vi "ATF-Hardware Config.vi"() -> ()   [LabVIEW 2022 SP3]
uses:
  Controls/SeCrTs-Config.ctl
panel:
  in  "Signal list":bool
  out "Config":T1={"AO config"=[], "AI config"=[], "DI config"=[], "DO config"=[], "TC config"=[{"Channel_Name"="", "Channel_Number"="", "Pre_Scale_min"=0.0, "Pre_Scale_max"=0.0, "units"=4, " type"=7}], "ACC config"=[], "SG config"=[], "Strain Gauge Settings"={"poisson ratio"=0.3, "nominal gage resistance"=120.0, "gage factor"=2.08}, "Bridge Settings"={"voltage excitation value"=3.3, "voltage excitation source"=10200, "initial bridge voltage"=0.0, "lead wire resistance"=1.7, "strain configuration"=10271}, "Sample Rate"={"AI Sample Rate"=[], "AO Sample Rate"=[], "DI Sample Rate"=[], "TC Sample Rate"=[], "DO Sample Rate"=[], "SG Sample Rate"=[], "ACC Sample Rate"=[]}} {"Bridge Settings"."strain configuration" items=["Full Bridge I"=10183, "Full Bridge II"=10184, "Full Bridge III"=10185, "Half Bridge I"=10188, "Half Bridge II"=10189, "Quarter Bridge I"=10271, "Quarter Bridge II"=10272]; "Bridge Settings"."voltage excitation source" items=["Internal"=10200, "External"=10167, "None"=10230]; "ACC config"."Terminal configuration" items=["default"=-1, "RSE"=10083, "NRSE"=10078, "Differential"=10106, "Pseudodifferential"=12529]; "ACC config"."Sensitivity units" items=["mVolts/g"=12509, "Volts/g"=12510]; "TC config"."type" items=["J"=10072, "K"=10073, "N"=10077, "R"=10082, "S"=10085, "T"=10086, "B"=10047, "E"=10055]; "TC config"."units" items=["Deg C", "Deg F", "Kelvins", "Deg R", "From Custom Scale"]}
  in  "Cancel":bool
  in  "Load Configuration":bool
  in  "New configuration":bool
  in  "Save Config":bool
  in  "Tab Control":T2(tab)
  in  "DO Sample Rate":dbl[](array[numeric]) format="%#_g Hz"
  in  "DO config":T3(array[cluster])=[{"Channel_Name"="", "Channel_Number"="", "Default_Value"=FALSE, "Units"=FALSE}]
  out "DO Device List":string[](array[string])
  in  "DI Sample Rate":dbl[](array[numeric]) format="%#_g Hz"
  in  "DI config":T3(array[cluster])
  out "DI Device List":string[](array[string])
  in  "AO Sample Rate":dbl[](array[numeric]) format="%#_g Hz"
  in  "AO config":T4(array[cluster])
  out "AO Device List":string[](array[string])
  in  "AI Sample Rate":dbl[](array[numeric]) format="%#_g Hz"
  in  "AI config":T5(array[cluster])
  out "AI Device List":string[](array[string])
  in  "TC Sample Rate":dbl[](array[numeric]) format="%#_g Hz"
  in  "TC config":T6(array[cluster]) {"thermocouple type" items=["J"=10072, "K"=10073, "N"=10077, "R"=10082, "S"=10085, "T"=10086, "B"=10047, "E"=10055]; "units" items=["Deg C"=10143, "Deg F"=10144, "Kelvins"=10325, "Deg R"=10145, "From Custom Scale"=10065]}
  out "TC Device List":string[](array[string])
  in  "ACC Sample Rate":dbl[](array[numeric]) format="%#_g Hz"
  in  "ACC config":T7(array[cluster]) {"Sensitivity units" items=["mVolts/g"=12509, "Volts/g"=12510]; "Terminal configuration" items=["default"=-1, "RSE"=10083, "NRSE"=10078, "Differential"=10106, "Pseudodifferential"=12529]}
  out "ACC Device List":string[](array[string])
  out "SG Device List":string[](array[string])
  in  "SG Sample Rate":dbl[](array[numeric]) format="%#_g Hz"
  in  "SG config":T8(array[cluster])
  in  "SG Settings":T9={"gage factor"=2.08, "nominal gage \nresistance"=120.0, "poisson ratio"=0.3}
  in  "Bridge Settings":T10={"voltage excitation value"=3.3, "voltage excitation source"=10200, "initial bridge voltage"=0.0, "lead wire resistance"=1.7, "strain configuration"=10271} {"strain configuration" items=["Full Bridge I"=10183, "Full Bridge II"=10184, "Full Bridge III"=10185, "Half Bridge I"=10188, "Half Bridge II"=10189, "Quarter Bridge I"=10271, "Quarter Bridge II"=10272]; "voltage excitation source" items=["Internal"=10200, "External"=10167, "None"=10230]}
  # "DO_Channel_Name"
  # "DO_Channel_Number"
  # "Default Value"
  # "Invert?"
  # "DI_Channel_Name"
  # "DI_Channel_Number"
  # "Default Value"
  # "Invert?"
  # "AO_Channel_Name"
  # "AO_Channel_Number"
  # "Default Value"
  # "Units"
  # "AI_Channel_Name"
  # "AI_Channel_Number"
  # "Pre_Scale_min"
  # "Pre_Scale_max"
  # "Scale_min"
  # "Scale_max"
  # "Units"
  # "TC_Channel_Name"
  # "TC_Channel_Number"
  # "Max_Value"
  # "Units"
  # "Type"
  # "Min_Value"
  # "ACC_Channel_Name"
  # "ACC_Channel_Number"
  # "Min_Value"
  # "Max_Value"
  # "Terminal Config"
  # "Sensitivity"
  # "Sensitivity Units"
  # "SG_Channel_Name"
  # "SG_Channel_Number"
  # "Min_Value"
  # "Max_Value"
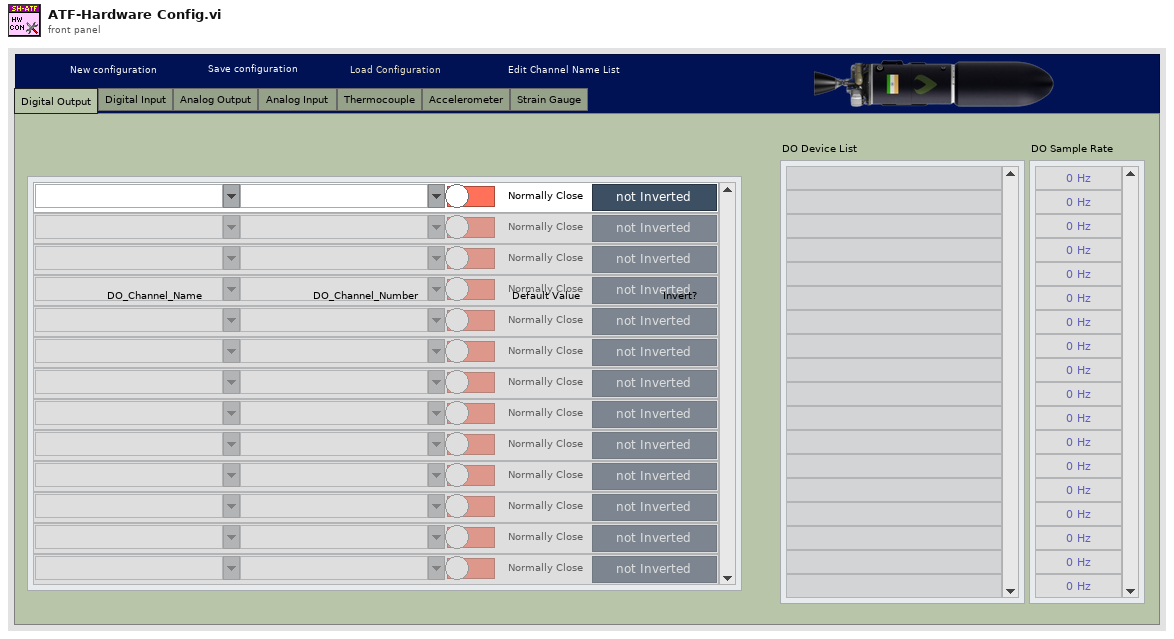
[diagram p1: front panel]
types:
  T1 = typedef "SeCrTs-Config.ctl" = cluster{"AO config":cluster{"Channel_Name":string, "Channel_Number":string, "Default_Value":dbl, "Units":string}[], "AI config":cluster{"Channel_Name":string, "Channel_Number":string, "Pre_Scale_min":dbl, "Pre_Scale_max":dbl, "Sensor_min":dbl, "Sensor_max":dbl, "Units":string}[], "DI config":cluster{"Channel_Name":string, "Channel_Number":string, "Default_Value":bool, "DI invert?":bool}[], "DO config":cluster{"Channel_Name":string, "Channel_Number":string, "Default_Value":bool, "DO invert?":bool}[], "TC config":cluster{"Channel_Name":string, "Channel_Number":string, "Pre_Scale_min":dbl, "Pre_Scale_max":dbl, "units":i32, " type":i32}[], "ACC config":cluster{"Channel_Name":string, "Channel_Number":string, "Pre_Scale_min":dbl, "Pre_Scale_max":dbl, "Terminal configuration":i32, "Sensitivity":dbl, "Sensitivity units":i32}[], "SG config":cluster{"Channel_Name":string, "Channel_Number":string, "Pre_Scale_min":dbl, "Pre_Scale_max":dbl}[], "Strain Gauge Settings":cluster{"poisson ratio":dbl, "nominal gage resistance":dbl, "gage factor":dbl}, "Bridge Settings":cluster{"voltage excitation value":dbl, "voltage excitation source":i32, "initial bridge voltage":dbl, "lead wire resistance":dbl, "strain configuration":i32}, "Sample Rate":cluster{"AI Sample Rate":dbl[], "AO Sample Rate":dbl[], "DI Sample Rate":dbl[], "TC Sample Rate":dbl[], "DO Sample Rate":dbl[], "SG Sample Rate":dbl[], "ACC Sample Rate":dbl[]}}
  T2 = enum32{"Digital Output", "Digital Input", "Analog Output", "Analog Input ", "Thermocouple", "Accelerometer", "Strain Gauge"}
  T3 = cluster{"Channel_Name":string, "Channel_Number":string, "Default_Value":bool, "Units":bool}[]
  T4 = cluster{"Channel_Name":string, "Channel_Number":string, "Default_Value":dbl, "Units":string}[]
  T5 = cluster{"Channel_Name":string, "Channel_Number":string, "Pre_Scale_min":dbl, "Pre_Scale_max":dbl, "Sensor_min":dbl, "Sensor_max":dbl, "Units":string}[]
  T6 = cluster{"Channel_Name":string, "Channel_Number":string, "Pre_Scale_min":dbl, "Pre_Scale_max":dbl, "units":i32, "thermocouple type":i32}[]
  T7 = cluster{"Channel_Name":string, "Channel_Number":string, "Pre_Scale_min":dbl, "Pre_Scale_max":dbl, "Terminal configuration":i32, "Sensitivity":dbl, "Sensitivity units":i32}[]
  T8 = cluster{"Channel_Name":string, "Channel_Number":string, "Pre_Scale_min":dbl, "Pre_Scale_max":dbl}[]
  T9 = cluster{"gage factor":dbl, "nominal gage \nresistance":dbl, "poisson ratio":dbl}
  T10 = cluster{"voltage excitation value":dbl, "voltage excitation source":i32, "initial bridge voltage":dbl, "lead wire resistance":dbl, "strain configuration":i32}
  T11 = cluster{"Device List":cluster{"AO Cards":tag[], "AI Cards":tag[], "DI Cards":tag[], "DO Cards":tag[]}, "Channel List":cluster{"AI Channel list":tag[], "AO Channel list":tag[], "DO Channel list ":tag[], "DI Channel list":tag[]}}
  T12 = cluster{"Channel List":cluster{"AI Channel list":tag[], "AO Channel list":tag[], "DO Channel list ":tag[], "DI Channel list":tag[]}, "Device List":cluster{"AO Cards":tag[], "AI Cards":tag[], "DI Cards":tag[], "DO Cards":tag[]}}
  T13 = cluster{"Data":T1, "path":path, "Name ref":refnum<vi>[], "Names":string[][], "Signal path":path, "SR":cluster{"AI Sample Rate":dbl[], "AO Sample Rate":dbl[], "DI Sample Rate":dbl[], "TC Sample Rate":dbl[], "DO Sample Rate":dbl[], "SG Sample Rate":dbl[], "ACC Sample Rate":dbl[]}, "Device List":cluster{"AO Cards":tag[], "AI Cards":tag[], "DI Cards":tag[], "DO Cards":tag[]}}
  T14 = typedef "SeCrTs-file folder ctl.ctl" = cluster{"Datalog path":path, "Configuration path":path, "Signal list path":path, "Sub vi's":path, "Authentication":path, "Sequence":path, "Event Log":path, "CS Error log":path, "RT Error Log":path}
  T15 = cluster{"AI":string[], "DI":string[], "DO":string[], "SG":string[], "AO":string[], "TC":string[], "ACC":string[]}
  T16 = cluster{"AI Channel list":tag[], "AO Channel list":tag[], "DO Channel list ":tag[], "DI Channel list":tag[]}
  T17 = cluster{"AO Cards":tag[], "AI Cards":tag[], "DI Cards":tag[], "DO Cards":tag[]}
  T18 = cluster{"AI Sample Rate":dbl[], "AO Sample Rate":dbl[], "DI Sample Rate":dbl[], "TC Sample Rate":dbl[], "DO Sample Rate":dbl[], "SG Sample Rate":dbl[], "ACC Sample Rate":dbl[]}
  T19 = enum16{"open", "replace", "create", "open or create", "replace or create", "replace or create with confirmation"}
  T20 = enum32{"Invalid", "Standard", "Closed", "Hidden", "Minimized", "Maximized"}
  T21 = cluster{"Channel_Name":string, "Channel_Number":string, "Default_Value":bool, "DI invert?":bool}[]
  T22 = cluster{"Channel_Name":string, "Channel_Number":string, "Default_Value":bool, "DO invert?":bool}[]
  T23 = cluster{"Channel_Name":string, "Channel_Number":string, "Pre_Scale_min":dbl, "Pre_Scale_max":dbl, "units":i32, " type":i32}[]
  T24 = cluster{"poisson ratio":dbl, "nominal gage resistance":dbl, "gage factor":dbl}
  T25 = cluster{"Channel_Name":string, "Channel_Number":string}
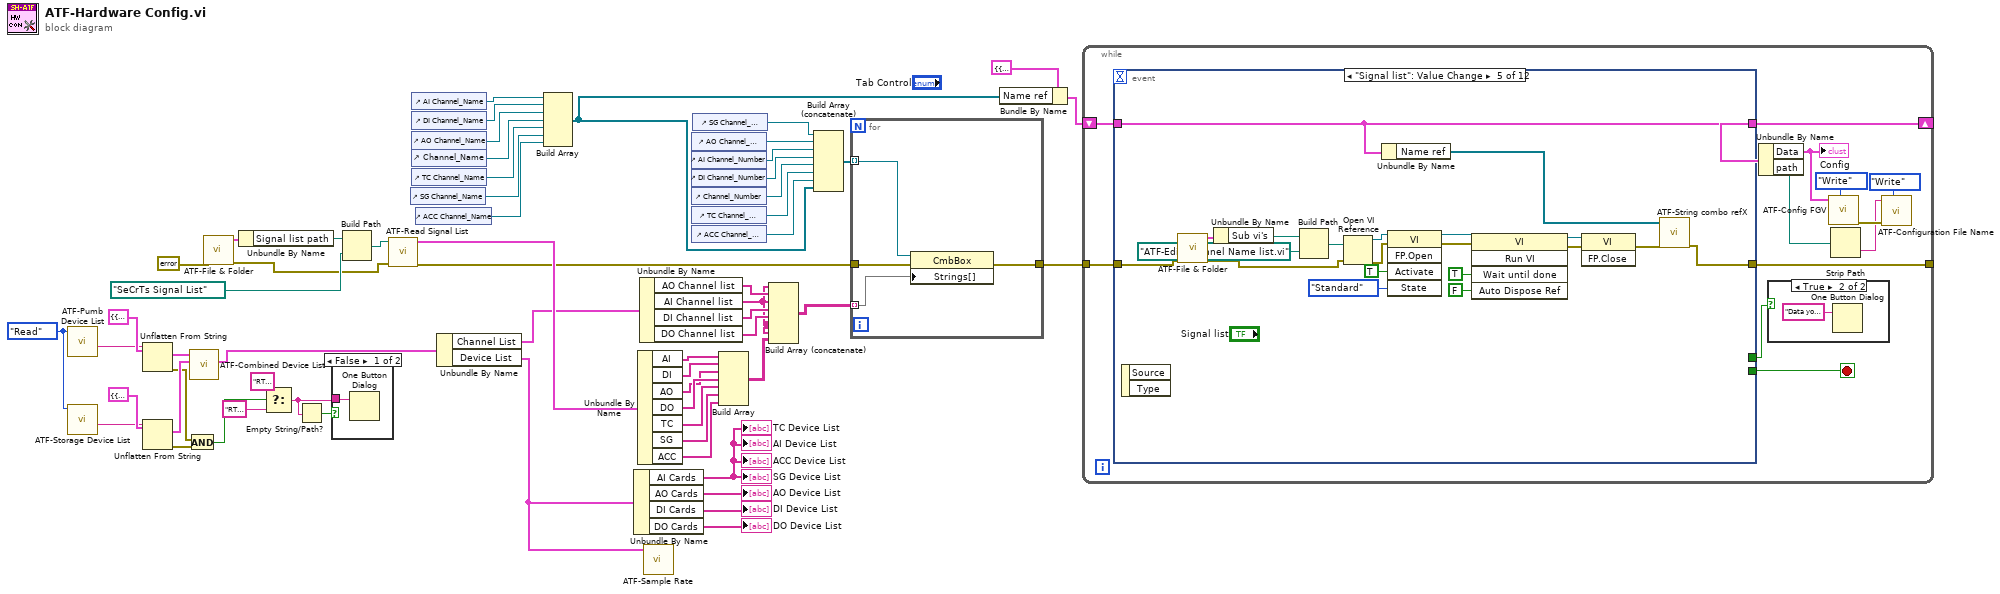
[diagram p0: block diagram]
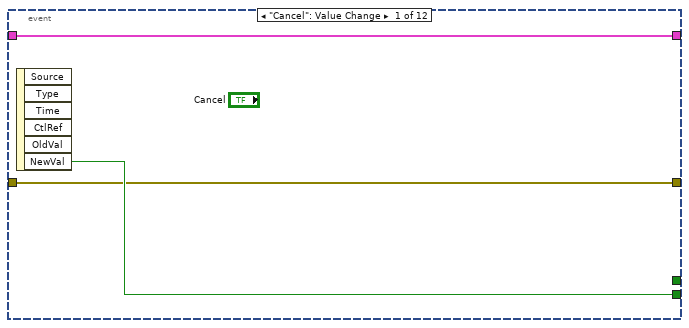
[diagram p4: hidden frame]
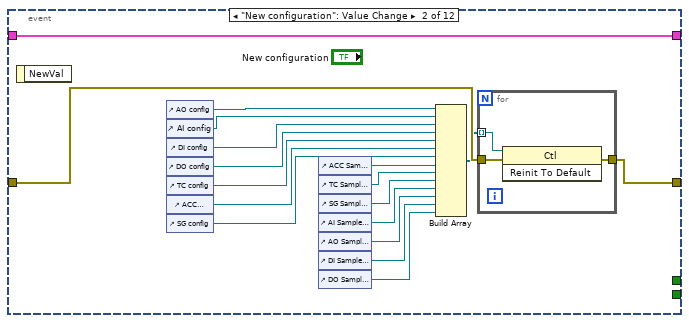
[diagram p5: hidden frame]
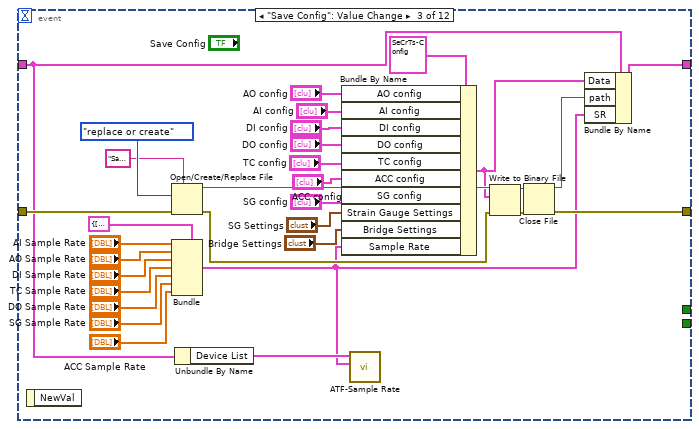
[diagram p6: hidden frame]
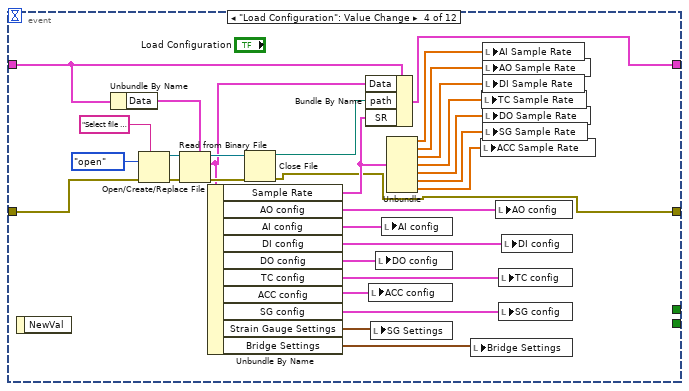
[diagram p7: hidden frame]
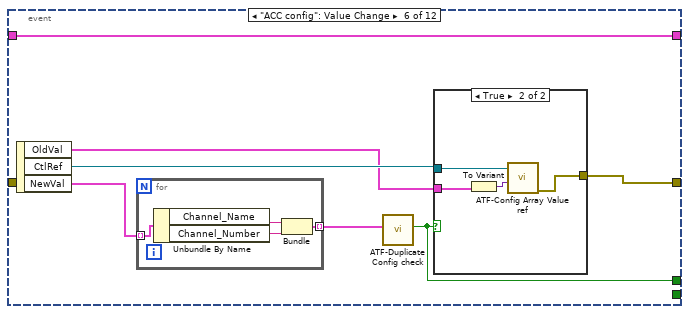
[diagram p8: hidden frame]
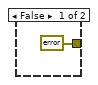
[diagram p9: hidden frame]
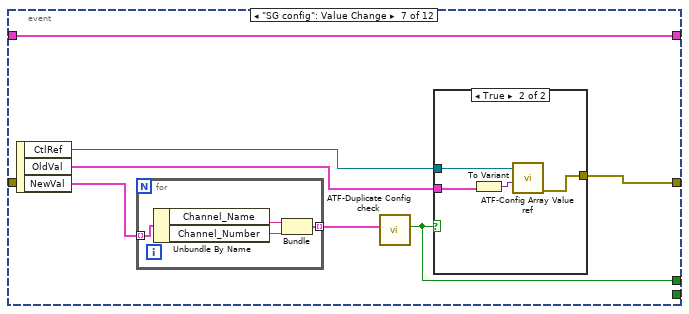
[diagram p10: hidden frame]
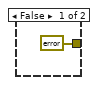
[diagram p11: hidden frame]
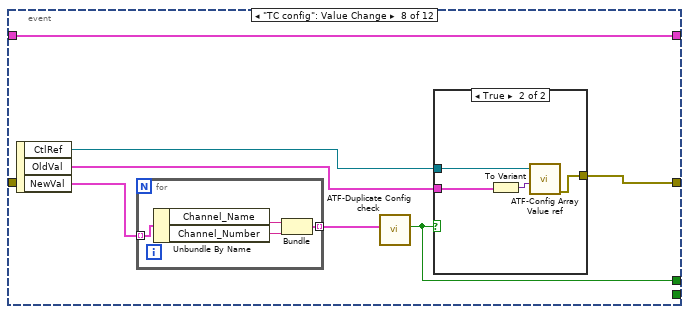
[diagram p12: hidden frame]
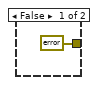
[diagram p13: hidden frame]
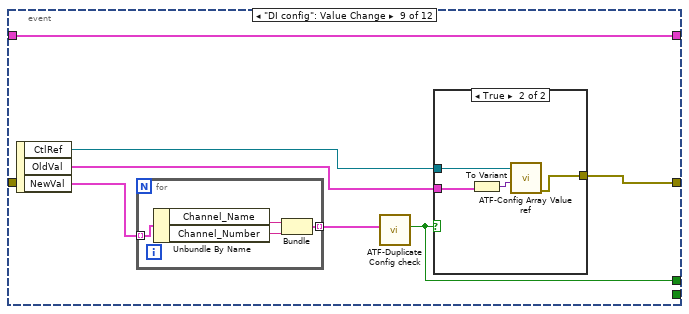
[diagram p14: hidden frame]
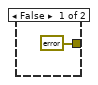
[diagram p15: hidden frame]
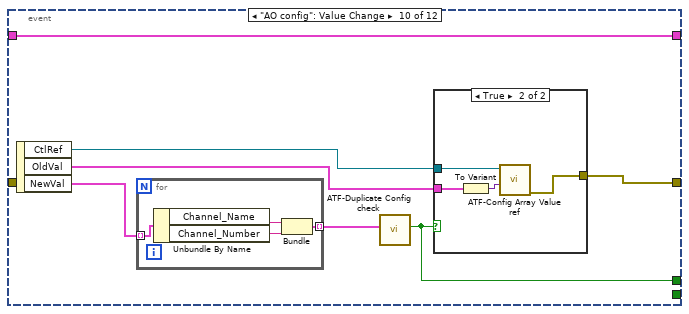
[diagram p16: hidden frame]
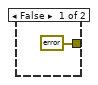
[diagram p17: hidden frame]
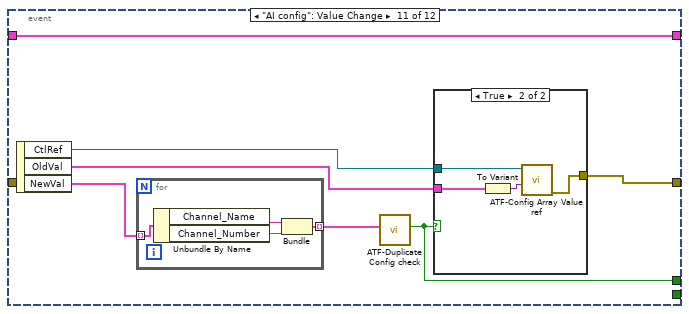
[diagram p18: hidden frame]
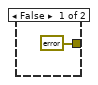
[diagram p19: hidden frame]
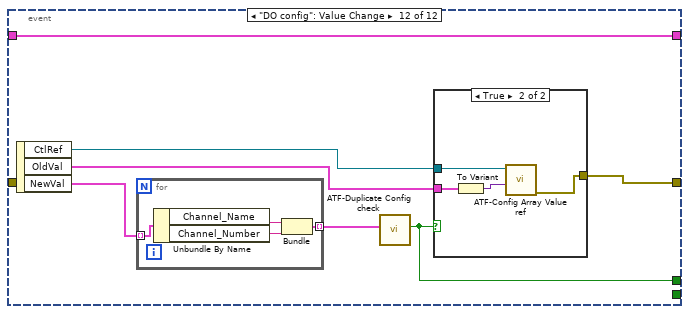
[diagram p20: hidden frame]
diagram:
  w14 = enum16{"Read", "Write", "Clear"}."Read" ("Enum")
  n1 = call "ATF-Pumb Device List.vi"("Enum"=w14) -> ("DL"=w3:string)  [unwired: 10 in]
  n2 = call "ATF-Storage Device List.vi"("Enum"=w14) -> ("DL"=w2:string)  [unwired: 10 in]
  n3 = Unflatten From String(type=T11 {"Device List"={"AO Cards"=[], "AI Cards"=[], "DI Cards"=[], "DO Cards"=[]}, "Channel List"={"AI Channel list"=[], "AO Channel list"=[], "DO Channel list "=[], "DI Channel list"=[]}}, binary string=w3) -> (value=w11:T11, error out=w6:errorcluster)  [unwired: 3 in, 1 out]
  n4 = Unflatten From String(type=T12 {"Channel List"={"AI Channel list"=[], "AO Channel list"=[], "DO Channel list "=[], "DI Channel list"=[]}, "Device List"={"AO Cards"=[], "AI Cards"=[], "DI Cards"=[], "DO Cards"=[]}}, binary string=w2) -> (value=w10:T12, error out=w5:errorcluster)  [unwired: 3 in, 1 out]
  n5 = And(x=w6, y=w5) -> (x .and. y?=w4:bool)
  n6 = call "ATF-Combined Device List.vi"("Storage"=w10, "Pump"=w11) -> ("Combined Device list"=w15:T12)  [unwired: 9 in]
  n7 = call "ATF-File & Folder.vi"("error in (no error)"=errorcluster {"status"=FALSE, "code"=0, "source"=""} ("error in")) -> ("error out"=w40:errorcluster, "File Output"=w46:T14)  [unwired: 9 in]
  n8 = Unbundle By Name(w46) -> ("Signal list path"=w45:path)
  n9 = Select(t="RT device list has not loaded!" ("DL"), s=w4, f="RT device list has been loaded.") -> (s? t:f=w7:string)
  n10 = Empty String/Path?(string/path=w7) -> (empty?=w9:bool)
  n11 = case shown="False" w9 {
    tunnel: w7 -> [w62 _]
    frame False {
      n12 = One Button Dialog(message=w62) -> ()  [unwired: 1 in, 1 out]
    }
    frame True {
    }
  }
  n13 = Build Path(base path=w45, name or relative path=path "SeCrTs Signal List") -> (appended path=w19:path)
  n14 = call "ATF-Read Signal List.vi"("error in"=w40, "file path (use dialog)"=w19) -> ("error out"=w18:errorcluster, "Names"=w39:T15)  [unwired: 8 in]
  n15 = control-ref of="SG Channel_Name"() -> (w25:refnum<vi>)
  n16 = control-ref of="AI Channel_Name"() -> (w43:refnum<vi>)
  n17 = control-ref of="DI Channel_Name"() -> (w42:refnum<vi>)
  n18 = control-ref of="AO Channel_Name"() -> (w27:refnum<vi>)
  n19 = control-ref of="Channel_Name"() -> (w26:refnum<vi>)
  n20 = control-ref of="TC Channel_Name"() -> (w41:refnum<vi>)
  n21 = control-ref of="ACC Channel_Name"() -> (w24:refnum<vi>)
  n22 = Unbundle By Name(w15) -> ("Channel List"=w16:T16, "Device List"=w17:T17)
  n23 = Build Array(w43, w42, w27, w26, w41, w25, w24) -> (w28:refnum<vi>[])
  n24 = Unbundle By Name(w17) -> ("AI Cards"=→"AI Device List" →"TC Device List" →"ACC Device List" →"SG Device List":tag[], "AO Cards"=→"AO Device List":tag[], "DI Cards"=→"DI Device List":tag[], "DO Cards"=→"DO Device List":tag[])
  n25 = Unbundle By Name(w39) -> ("AI"=w38:string[], "DI"=w37:string[], "AO"=w32:string[], "DO"=w36:string[], "TC"=w35:string[], "SG"=w34:string[], "ACC"=w33:string[])
  n26 = Unbundle By Name(w16) -> ("AO Channel list"=w49:tag[], "AI Channel list"=w48:tag[], "DI Channel list"=w56:tag[], "DO Channel list"=w55:tag[])
  n27 = call "ATF-Sample Rate.vi"("Device List"=w17) -> ()  [unwired: 11 in]
  n28 = control-ref of="AO Channel_Number"() -> (w61:refnum<vi>)
  n29 = control-ref of="AI Channel_Number"() -> (w60:refnum<vi>)
  n30 = control-ref of="DI Channel_Number"() -> (w59:refnum<vi>)
  n31 = control-ref of="Channel_Number"() -> (w58:refnum<vi>)
  n32 = control-ref of="TC Channel_Number"() -> (w52:refnum<vi>)
  n33 = control-ref of="ACC Channel_Number"() -> (w51:refnum<vi>)
  n34 = control-ref of="SG Channel_Number"() -> (w50:refnum<vi>)
  n35 = Build Array(w38, w37, w32, w36, w35, w34, w33) -> (w31:string[][])
  n36 = Build Array (concatenate)(w48, w49, w48, w56, w55, w48, w48, w31) -> (w54:string[][])
  n37 = Build Array (concatenate)(w50, w61, w60, w59, w58, w52, w51, w28) -> (w57:refnum<vi>[])
  n38 = for {
    tunnel: w57 -> [w66] mode=indexing
    tunnel: w54 -> [w63] mode=indexing
    tunnel: [w65] -> w53
    tunnel: w18 -> [w64]
    n39 = property class="CmbBox"(reference=w66, error in=w64, "Strings[]"=w63) -> (error out=w65:errorcluster)  [unwired: 1 out]
  }
  n40 = Bundle By Name(cluster=T13 {"Data"={"AO config"=[], "AI config"=[], "DI config"=[], "DO config"=[], "TC config"=[{"Channel_Name"="", "Channel_Number"="", "Pre_Scale_min"=0.0, "Pre_Scale_max"=0.0, "units"=4, " type"=7}], "ACC config"=[], "SG config"=[], "Strain Gauge Settings"={"poisson ratio"=0.3, "nominal gage resistance"=120.0, "gage factor"=2.08}, "Bridge Settings"={"voltage excitation value"=3.3, "voltage excitation source"=10200, "initial bridge voltage"=0.0, "lead wire resistance"=1.7, "strain configuration"=10271}, "Sample Rate"={"AI Sample Rate"=[], "AO Sample Rate"=[], "DI Sample Rate"=[], "TC Sample Rate"=[], "DO Sample Rate"=[], "SG Sample Rate"=[], "ACC Sample Rate"=[]}}, "path"=path "", "Name ref"=[], "Names"=[], "Signal path"=path "", "SR"={"AI Sample Rate"=[], "AO Sample Rate"=[], "DI Sample Rate"=[], "TC Sample Rate"=[], "DO Sample Rate"=[], "SG Sample Rate"=[], "ACC Sample Rate"=[]}, "Device List"={"AO Cards"=["PXI1Slot2"], "AI Cards"=["cDAQ1Mod1", "cDAQ1Mod2", "cDAQ1Mod3", "cDAQ1Mod4"], "DI Cards"=["cDAQ1Mod5", "PXI1Slot2", "PXI1Slot3"], "DO Cards"=["cDAQ1Mod5", "PXI1Slot2", "PXI1Slot3"]}}, "Name ref"=w28) -> (w30:T13)
  n41 = while {
    shift-right: [w74] -> _
    shift-left: w30 -> [w75]
    tunnel: w53 -> [w77]
    tunnel: [w76] -> _
    stop <- w78 stop-if-true
    n42 = event shown="[4] \"Signal list\": Value Change" {
      selector: _ -> [_ _ _ _ _ _ _ _ _ _ _ _]
      dyn-events: _ -> [_ _ _ _ _ _ _ _ _ _ _ _]
      timeout: _ -> [_ _ _ _ _ _ _ _ _ _ _ _]
      tunnel: [w81 _ _ _ _ _ _ _ _ _ _ _] -> w78
      tunnel: w77 -> [w80 w100 w135 w165 w185 _ _ _ _ _ _ _]
      tunnel: [w80 w99 w131 w142 w167 w187 w205 w221 w237 w253 w269 w285] -> w76
      tunnel: w75 -> [w82 w98 w107 w156 w170 w192 w208 w224 w240 w256 w272 w288]
      tunnel: [w82 w98 w123 w157 w170 w192 w208 w224 w240 w256 w272 w288] -> w74
      tunnel: [_ _ _ _ _ w186 w202 w218 w234 w250 w266 w282] -> w70
      event "Cancel": Value Change {
        n43 = event-data() -> ("NewVal"=w81:bool)  [unwired: 1 in, 5 out]
      }
      event "New configuration": Value Change {
        n44 = event-data() -> ()  [unwired: 1 in, 1 out]
        n45 = control-ref of="AO config"() -> (w93:refnum<vi>)
        n46 = control-ref of="AI config"() -> (w94:refnum<vi>)
        n47 = control-ref of="DI config"() -> (w95:refnum<vi>)
        n48 = control-ref of="DO config"() -> (w96:refnum<vi>)
        n49 = control-ref of="TC config"() -> (w92:refnum<vi>)
        n50 = control-ref of="ACC config"() -> (w91:refnum<vi>)
        n51 = control-ref of="SG config"() -> (w90:refnum<vi>)
        n52 = control-ref of="ACC Sample Rate"() -> (w89:refnum<vi>)
        n53 = control-ref of="TC Sample Rate"() -> (w88:refnum<vi>)
        n54 = control-ref of="SG Sample Rate"() -> (w87:refnum<vi>)
        n55 = control-ref of="AI Sample Rate"() -> (w86:refnum<vi>)
        n56 = control-ref of="AO Sample Rate"() -> (w85:refnum<vi>)
        n57 = control-ref of="DI Sample Rate"() -> (w84:refnum<vi>)
        n58 = control-ref of="DO Sample Rate"() -> (w83:refnum<vi>)
        n59 = Build Array(w93, w94, w95, w96, w92, w91, w90, w89, w88, w87, w86, w85, w84, w83) -> (w97:refnum<vi>[])
        n60 = for {
          tunnel: w97 -> [w103] mode=indexing
          tunnel: w100 -> [w102]
          tunnel: [w101] -> w99
          n61 = invoke class="Ctl" method="Reinit To Default"(reference=w103, error in=w102) -> (error out=w101:errorcluster)  [unwired: 1 in, 2 out]
        }
      }
      event "Save Config": Value Change {
        n62 = event-data() -> ()  [unwired: 1 in, 1 out]
        n63 = Open/Create/Replace File(error in=w135, prompt="Save Changes", operation (0:open)=T19."replace or create") -> (refnum out=w130:refnum<file>, error out=w134:errorcluster)  [unwired: 3 in, 1 out]
        n64 = Bundle(cluster=T18 {"AI Sample Rate"=[], "AO Sample Rate"=[], "DI Sample Rate"=[], "TC Sample Rate"=[], "DO Sample Rate"=[], "SG Sample Rate"=[], "ACC Sample Rate"=[]} ("Sample Rate"), "AI Sample Rate"="AI Sample Rate", "AO Sample Rate"="AO Sample Rate", "DI Sample Rate"="DI Sample Rate", "TC Sample Rate"="TC Sample Rate", "DO Sample Rate"="DO Sample Rate", "SG Sample Rate"="SG Sample Rate", "ACC Sample Rate"="ACC Sample Rate") -> (w105:T18)
        n65 = Unbundle By Name(w107) -> ("Device List"=w106:T17)
        n66 = Bundle By Name(cluster=T1 {"AO config"=[], "AI config"=[], "DI config"=[], "DO config"=[], "TC config"=[{"Channel_Name"="", "Channel_Number"="", "Pre_Scale_min"=0.0, "Pre_Scale_max"=0.0, "units"=4, " type"=7}], "ACC config"=[], "SG config"=[], "Strain Gauge Settings"={"poisson ratio"=0.3, "nominal gage resistance"=120.0, "gage factor"=2.08}, "Bridge Settings"={"voltage excitation value"=3.3, "voltage excitation source"=10200, "initial bridge voltage"=0.0, "lead wire resistance"=1.7, "strain configuration"=10271}, "Sample Rate"={"AI Sample Rate"=[], "AO Sample Rate"=[], "DI Sample Rate"=[], "TC Sample Rate"=[], "DO Sample Rate"=[], "SG Sample Rate"=[], "ACC Sample Rate"=[]}} ("Data"), "AO config"="AO config", "AI config"="AI config", "DI config"="DI config", "DO config"="DO config", "TC config"="TC config", "ACC config"="ACC config", "SG config"="SG config", "Strain Gauge Settings"="SG Settings", "Bridge Settings"="Bridge Settings", "Sample Rate"=w105) -> (w104:T1)
        n67 = call "ATF-Sample Rate.vi"("Sample Rate"=w105, "Device List"=w106) -> ()  [unwired: 10 in]
        n68 = Write to Binary File(file (use dialog)=w130, data=w104, error in=w134) -> (refnum out=w133:refnum<file>, error out=w132:errorcluster)  [unwired: 3 in, 1 out]
        n69 = Close File(refnum=w133, error in=w132) -> (path=w118:path, error out=w131:errorcluster)
        n70 = Bundle By Name(cluster=w107, "Data"=w104, "path"=w118, "SR"=w105) -> (w123:T13)
      }
      event "Load Configuration": Value Change {
        n71 = event-data() -> ()  [unwired: 1 in, 1 out]
        n72 = Unbundle By Name(w156) -> ("Data"=w158:T1)
        n73 = Open/Create/Replace File(error in=w165, prompt="Select file to load", operation (0:open)=T19."open") -> (refnum out=w161:refnum<file>, error out=w164:errorcluster)  [unwired: 3 in, 1 out]
        n74 = Read from Binary File(5:w158, 8:w164, 11:w161) -> (0:w162:errorcluster, 2:w155:T1, 3:w163:refnum<file>)  [unwired: 3 in, 1 out]
        n75 = Unbundle By Name(w155) -> ("Sample Rate"=w144:T18, "AO config"=w154:T4, "AI config"=w153:T5, "DI config"=w152:T21, "DO config"=w151:T22, "TC config"=w150:T23, "ACC config"=w149:T7, "SG config"=w148:T8, "Strain Gauge Settings"=w146:T24, "Bridge Settings"=w145:T10)
        n76 = Close File(refnum=w163, error in=w162) -> (path=w147:path, error out=w142:errorcluster)
        n77 = Bundle By Name(cluster=w156, "Data"=w155, "path"=w147, "SR"=w144) -> (w157:T13)
        n78 = local write "ACC config"(w149) -> ()
        n79 = local write "SG Settings"(w146) -> ()
        n80 = local write "DO config"(w151) -> ()
        n81 = local write "AI config"(w153) -> ()
        n82 = Unbundle(w144) -> ("AI Sample Rate"=w143:dbl[], "AO Sample Rate"=w141:dbl[], "DI Sample Rate"=w140:dbl[], "TC Sample Rate"=w139:dbl[], "DO Sample Rate"=w138:dbl[], "SG Sample Rate"=w137:dbl[], "ACC Sample Rate"=w136:dbl[])
        n83 = local write "Bridge Settings"(w145) -> ()
        n84 = local write "ACC Sample Rate"(w136) -> ()
        n85 = local write "TC Sample Rate"(w139) -> ()
        n86 = local write "AI Sample Rate"(w143) -> ()
        n87 = local write "AO Sample Rate"(w141) -> ()
        n88 = local write "DI Sample Rate"(w140) -> ()
        n89 = local write "DO Sample Rate"(w138) -> ()
        n90 = local write "SG Sample Rate"(w137) -> ()
        n91 = local write "AO config"(w154) -> ()
        n92 = local write "TC config"(w150) -> ()
        n93 = local write "SG config"(w148) -> ()
        n94 = local write "DI config"(w152) -> ()
      }
      event "Signal list": Value Change {
        n95 = event-data() -> ()  [unwired: 1 in, 2 out]
        n96 = call "ATF-File & Folder.vi"("error in (no error)"=w185) -> ("error out"=w181:errorcluster, "File Output"=w184:T14)  [unwired: 9 in]
        n97 = Unbundle By Name(w184) -> ("Sub vi's"=w183:path)
        n98 = Build Path(base path=w183, name or relative path=path "ATF-Edit Channel Name list.vi") -> (appended path=w166:path)
        n99 = Open VI Reference(vi path=w166, error in (no error)=w181) -> (vi reference=w172:refnum<vi>, error out=w171:errorcluster)  [unwired: 4 in]
        n100 = Unbundle By Name(w170) -> ("Name ref"=w169:refnum<vi>[])
        n101 = invoke class="VI" method="FP.Open"(reference=w172, error in=w171, "Activate"=TRUE ("Activate?"), "State"=T20."Standard") -> (reference out=w180:refnum<vi>, error out=w179:errorcluster)  [unwired: 1 in, 3 out]
        n102 = invoke class="VI" method="Run VI"(reference=w180, error in=w179, "Wait until done"=TRUE ("Wait Until Done"), "Auto Dispose Ref"=FALSE ("Auto Dispose Reference")) -> (reference out=w178:refnum<vi>, error out=w177:errorcluster)  [unwired: 1 in, 3 out]
        n103 = invoke class="VI" method="FP.Close"(reference=w178, error in=w177) -> (error out=w168:errorcluster)  [unwired: 1 in, 2 out]
        n104 = call "ATF-String combo refX.vi"("error out"=w168, "Ctrl ref"=w169) -> ("error out 2"=w167:errorcluster)  [unwired: 9 in]
      }
      event "ACC config": Value Change {
        n105 = event-data() -> ("OldVal"=w188:T7, "CtlRef"=w189:refnum<vi>, "NewVal"=w191:T7)  [unwired: 1 in]
        n106 = for {
          tunnel: w191 -> [w196] mode=indexing
          tunnel: [w193] -> w190 mode=indexing
          n107 = Unbundle By Name(w196) -> ("Channel_Name"=w194:string, "Channel_Number"=w195:string)
          n108 = Bundle("Channel_Name"=w194, "Channel_Number"=w195) -> (w193:T25)  [unwired: 1 in]
        }
        n109 = call "ATF-Duplicate Config check.vi"("Data in"=w190) -> ("Channel list indication"=w186:bool)  [unwired: 10 in]
        n110 = case shown="True" w186 {
          tunnel: w189 -> [_ w200]
          tunnel: w188 -> [_ w199]
          tunnel: [errorcluster {"status"=FALSE, "code"=0, "source"=""} ("error out") w198] -> w187
          frame False {
          }
          frame True {
            n111 = To Variant(anything=w199) -> (Variant=w201:variant)
            n112 = call "ATF-Config Array Value ref.vi"("Value"=w201, "Array in"=w200) -> ("error out"=w198:errorcluster)  [unwired: 9 in]
          }
        }
      }
      event "SG config": Value Change {
        n113 = event-data() -> ("CtlRef"=w204:refnum<vi>, "OldVal"=w203:T8, "NewVal"=w207:T8)  [unwired: 1 in]
        n114 = for {
          tunnel: w207 -> [w212] mode=indexing
          tunnel: [w209] -> w206 mode=indexing
          n115 = Unbundle By Name(w212) -> ("Channel_Name"=w210:string, "Channel_Number"=w211:string)
          n116 = Bundle("Channel_Name"=w210, "Channel_Number"=w211) -> (w209:T25)  [unwired: 1 in]
        }
        n117 = call "ATF-Duplicate Config check.vi"("Data in"=w206) -> ("Channel list indication"=w202:bool)  [unwired: 10 in]
        n118 = case shown="True" w202 {
          tunnel: w204 -> [_ w216]
          tunnel: w203 -> [_ w215]
          tunnel: [errorcluster {"status"=FALSE, "code"=0, "source"=""} ("error out") w214] -> w205
          frame False {
          }
          frame True {
            n119 = To Variant(anything=w215) -> (Variant=w217:variant)
            n120 = call "ATF-Config Array Value ref.vi"("Value"=w217, "Array in"=w216) -> ("error out"=w214:errorcluster)  [unwired: 9 in]
          }
        }
      }
      event "TC config": Value Change {
        n121 = event-data() -> ("CtlRef"=w220:refnum<vi>, "OldVal"=w219:T6, "NewVal"=w223:T6)  [unwired: 1 in]
        n122 = for {
          tunnel: w223 -> [w228] mode=indexing
          tunnel: [w225] -> w222 mode=indexing
          n123 = Unbundle By Name(w228) -> ("Channel_Name"=w226:string, "Channel_Number"=w227:string)
          n124 = Bundle("Channel_Name"=w226, "Channel_Number"=w227) -> (w225:T25)  [unwired: 1 in]
        }
        n125 = call "ATF-Duplicate Config check.vi"("Data in"=w222) -> ("Channel list indication"=w218:bool)  [unwired: 10 in]
        n126 = case shown="True" w218 {
          tunnel: w220 -> [_ w232]
          tunnel: w219 -> [_ w231]
          tunnel: [errorcluster {"status"=FALSE, "code"=0, "source"=""} ("error out") w230] -> w221
          frame False {
          }
          frame True {
            n127 = To Variant(anything=w231) -> (Variant=w233:variant)
            n128 = call "ATF-Config Array Value ref.vi"("Value"=w233, "Array in"=w232) -> ("error out"=w230:errorcluster)  [unwired: 9 in]
          }
        }
      }
      event "DI config": Value Change {
        n129 = event-data() -> ("CtlRef"=w236:refnum<vi>, "OldVal"=w235:T3, "NewVal"=w239:T3)  [unwired: 1 in]
        n130 = for {
          tunnel: w239 -> [w244] mode=indexing
          tunnel: [w241] -> w238 mode=indexing
          n131 = Unbundle By Name(w244) -> ("Channel_Name"=w242:string, "Channel_Number"=w243:string)
          n132 = Bundle("Channel_Name"=w242, "Channel_Number"=w243) -> (w241:T25)  [unwired: 1 in]
        }
        n133 = call "ATF-Duplicate Config check.vi"("Data in"=w238) -> ("Channel list indication"=w234:bool)  [unwired: 10 in]
        n134 = case shown="True" w234 {
          tunnel: w236 -> [_ w248]
          tunnel: w235 -> [_ w247]
          tunnel: [errorcluster {"status"=FALSE, "code"=0, "source"=""} ("error out") w246] -> w237
          frame False {
          }
          frame True {
            n135 = To Variant(anything=w247) -> (Variant=w249:variant)
            n136 = call "ATF-Config Array Value ref.vi"("Value"=w249, "Array in"=w248) -> ("error out"=w246:errorcluster)  [unwired: 9 in]
          }
        }
      }
      event "AO config": Value Change {
        n137 = event-data() -> ("CtlRef"=w252:refnum<vi>, "OldVal"=w251:T4, "NewVal"=w255:T4)  [unwired: 1 in]
        n138 = for {
          tunnel: w255 -> [w260] mode=indexing
          tunnel: [w257] -> w254 mode=indexing
          n139 = Unbundle By Name(w260) -> ("Channel_Name"=w258:string, "Channel_Number"=w259:string)
          n140 = Bundle("Channel_Name"=w258, "Channel_Number"=w259) -> (w257:T25)  [unwired: 1 in]
        }
        n141 = call "ATF-Duplicate Config check.vi"("Data in"=w254) -> ("Channel list indication"=w250:bool)  [unwired: 10 in]
        n142 = case shown="True" w250 {
          tunnel: w252 -> [_ w265]
          tunnel: w251 -> [_ w263]
          tunnel: [errorcluster {"status"=FALSE, "code"=0, "source"=""} ("error out") w264] -> w253
          frame False {
          }
          frame True {
            n143 = To Variant(anything=w263) -> (Variant=w262:variant)
            n144 = call "ATF-Config Array Value ref.vi"("Value"=w262, "Array in"=w265) -> ("error out"=w264:errorcluster)  [unwired: 9 in]
          }
        }
      }
      event "AI config": Value Change {
        n145 = event-data() -> ("CtlRef"=w268:refnum<vi>, "OldVal"=w267:T5, "NewVal"=w271:T5)  [unwired: 1 in]
        n146 = for {
          tunnel: w271 -> [w276] mode=indexing
          tunnel: [w273] -> w270 mode=indexing
          n147 = Unbundle By Name(w276) -> ("Channel_Name"=w274:string, "Channel_Number"=w275:string)
          n148 = Bundle("Channel_Name"=w274, "Channel_Number"=w275) -> (w273:T25)  [unwired: 1 in]
        }
        n149 = call "ATF-Duplicate Config check.vi"("Data in"=w270) -> ("Channel list indication"=w266:bool)  [unwired: 10 in]
        n150 = case shown="True" w266 {
          tunnel: w268 -> [_ w280]
          tunnel: w267 -> [_ w279]
          tunnel: [errorcluster {"status"=FALSE, "code"=0, "source"=""} ("error out") w278] -> w269
          frame False {
          }
          frame True {
            n151 = To Variant(anything=w279) -> (Variant=w281:variant)
            n152 = call "ATF-Config Array Value ref.vi"("Value"=w281, "Array in"=w280) -> ("error out"=w278:errorcluster)  [unwired: 9 in]
          }
        }
      }
      event "DO config": Value Change {
        n153 = event-data() -> ("CtlRef"=w284:refnum<vi>, "OldVal"=w283:T3, "NewVal"=w287:T3)  [unwired: 1 in]
        n154 = for {
          tunnel: w287 -> [w292] mode=indexing
          tunnel: [w289] -> w286 mode=indexing
          n155 = Unbundle By Name(w292) -> ("Channel_Name"=w290:string, "Channel_Number"=w291:string)
          n156 = Bundle("Channel_Name"=w290, "Channel_Number"=w291) -> (w289:T25)  [unwired: 1 in]
        }
        n157 = call "ATF-Duplicate Config check.vi"("Data in"=w286) -> ("Channel list indication"=w282:bool)  [unwired: 10 in]
        n158 = case shown="True" w282 {
          tunnel: w284 -> [_ w297]
          tunnel: w283 -> [_ w295]
          tunnel: [errorcluster {"status"=FALSE, "code"=0, "source"=""} ("error out") w296] -> w285
          frame False {
          }
          frame True {
            n159 = To Variant(anything=w295) -> (Variant=w294:variant)
            n160 = call "ATF-Config Array Value ref.vi"("Value"=w294, "Array in"=w297) -> ("error out"=w296:errorcluster)  [unwired: 9 in]
          }
        }
      }
    }
    n161 = Unbundle By Name(w74) -> ("Data"=w73:T1, "path"=w71:path)
    "Config" <- w73
    n162 = case shown="True" w70 {
      frame False {
      }
      frame True {
        n163 = One Button Dialog ("Warning")(message="Data you Entered is already Exist!") -> ()  [unwired: 1 in, 1 out]
      }
    }
    n164 = call "ATF-Config FGV.vi"("Enum"=enum16{"Read", "Write"}."Write", "Data 2"=w73) -> ("error out"=w69:errorcluster)  [unwired: 8 in, 1 out]
    n165 = Strip Path(path=w71) -> (name=w68:string)  [unwired: 1 out]
    n166 = call "ATF-Configuration File Name.vi"("Enum"=enum16{"Read", "Write"}."Write", "error in"=w69, "Phase code W"=w68) -> ()  [unwired: 7 in, 2 out]
  }
